vi "SwTmr Get Scale Labels.vi"(11 "Array of Waveforms":waveform(dbl)[](array[waveform])) -> (1 "Y Scale Label Text":string, 2 "X Scale Label Text":string)   [LabVIEW 2017]
doc: "Returns the scale labels of the first waveform in the array of waveforms. If a scale is not specified in the waveform attributes returns Time and Amplitude as the X and Y labels respectively."
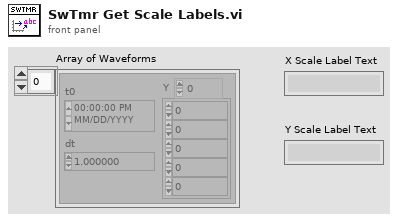
[diagram p1: front panel]
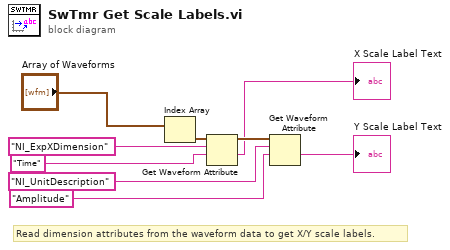
[diagram p0: block diagram]
diagram:
  # "Read dimension attributes from the waveform data to get X/Y scale labels."
  n1 = Index Array(array="Array of Waveforms") -> (element=w2:waveform(dbl))  [unwired: 1 in]
  n2 = Get Waveform Attribute(5:"Time" ("Time"), 6:"NI_ExpXDimension", 7:w2) -> (1:→"X Scale Label Text":string, 3:w5:waveform(dbl))  [unwired: 1 in, 2 out]
  n3 = Get Waveform Attribute(5:"Amplitude" ("Amplitude"), 6:"NI_UnitDescription", 7:w5) -> (1:→"Y Scale Label Text":string)  [unwired: 1 in, 3 out]
